vi "Page_Info_Initialize.vi"(8 "error in (no error)":errorcluster, 9 "ctlReferences":T1, 11 "AB_InteropAssembly in":refnum<class "AB_InteropAssembly.lvclass">) -> (0 "error out":errorcluster, 3 "AB_InteropAssembly out":refnum<class "AB_InteropAssembly.lvclass">)   [LabVIEW 2020, in "AB_InteropAssembly.lvclass"]
uses:
  <vilib>/AppBuilder/AB_Classes/InteropAssembly/AB_InteropAssembly.lvclass
  <resource>/Framework/Providers/Builds/AppBuilder/AB_UI_Page_Info_References.ctl
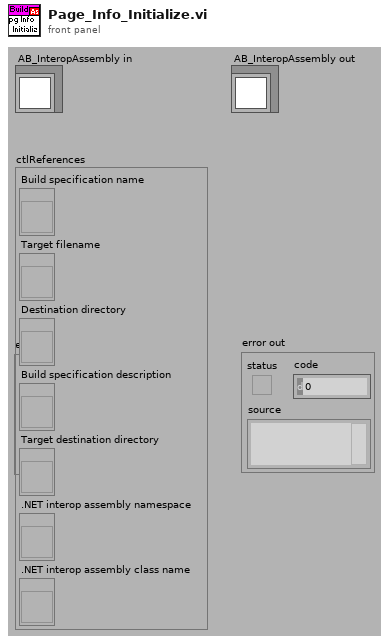
[diagram p1: front panel]
types:
  T1 = typedef "AB_UI_Page_Info_References.ctl" = cluster{"Build specification name":refnum<vi>, "Target filename":refnum<vi>, "Destination directory":refnum<vi>, "Build specification description":refnum<vi>, "Target destination directory":refnum<vi>, ".NET interop assembly namespace":refnum<vi>, ".NET interop assembly class name":refnum<vi>}
  T2 = typedef "LVRectTypeDef.ctl" = cluster{"Left":i16, "Top":i16, "Right":i16, "Bottom":i16}
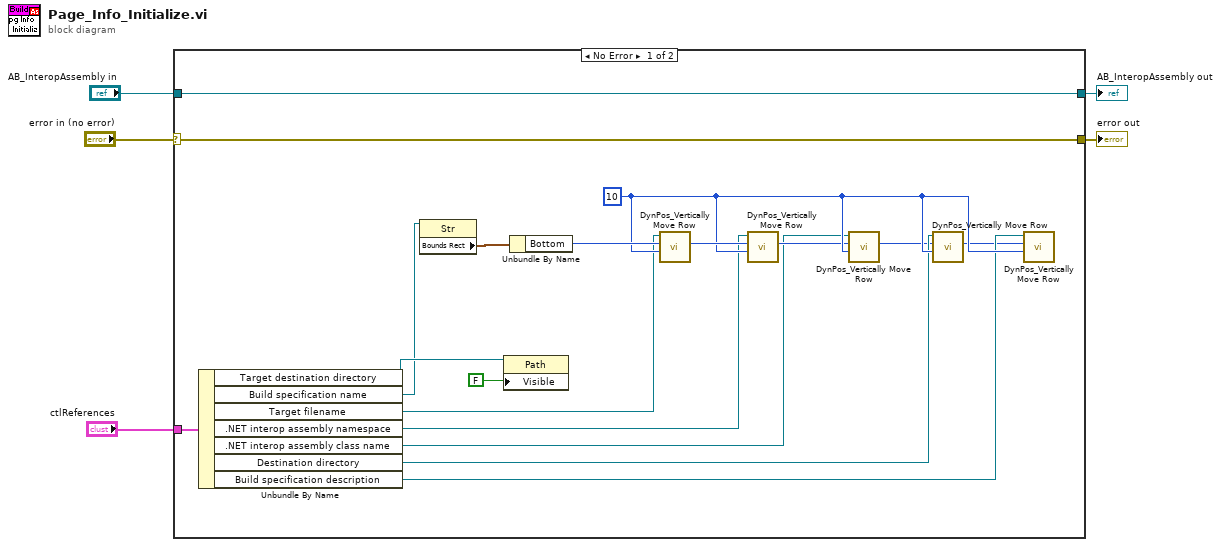
[diagram p0: block diagram]
diagram:
  n1 = case shown="No Error" "error in (no error)" {
    selector: "error in (no error)" -> [w6 w25]
    tunnel: [w6 w25] -> w1
    tunnel: [w7 w24] -> w4
    tunnel: "AB_InteropAssembly in" -> [w7 w24]
    tunnel: "ctlReferences" -> [w16 _]
    frame No Error {
      w17 = 10 ("Pixel separation (6)")
      n2 = Unbundle By Name(w16) -> ("Target destination directory"=w19:refnum<vi>, "Build specification name"=w18:refnum<vi>, "Target filename"=w13:refnum<vi>, ".NET interop assembly namespace"=w8:refnum<vi>, ".NET interop assembly class name"=w9:refnum<vi>, "Destination directory"=w14:refnum<vi>, "Build specification description"=w15:refnum<vi>)
      n3 = property class="Str"(reference=w18) -> ("Bounds Rect"=w23:T2)  [unwired: 1 in, 2 out]
      n4 = property class="Path"(reference=w19, "Visible"=FALSE) -> ()  [unwired: 1 in, 2 out]
      n5 = Unbundle By Name(w23) -> ("Bottom"=w22:i16)
      n6 = call <vilib>:"DynPos_Vertically Move Row.vi"("Pixel separation (6)"=w17, "Bottom of last control"=w22, "Control"=w13) -> ("Bottom pixel"=w21:i32)  [unwired: 1 in, 7 out]
      n7 = call <vilib>:"DynPos_Vertically Move Row.vi"("Pixel separation (6)"=w17, "Bottom of last control"=w21, "Control"=w8) -> ("Bottom pixel"=w12:i32)  [unwired: 1 in, 7 out]
      n8 = call <vilib>:"DynPos_Vertically Move Row.vi"("Pixel separation (6)"=w17, "Bottom of last control"=w12, "Control"=w9) -> ("Bottom pixel"=w11:i32)  [unwired: 1 in, 7 out]
      n9 = call <vilib>:"DynPos_Vertically Move Row.vi"("Pixel separation (6)"=w17, "Bottom of last control"=w11, "Control"=w14) -> ("Bottom pixel"=w10:i32)  [unwired: 1 in, 7 out]
      n10 = call <vilib>:"DynPos_Vertically Move Row.vi"("Pixel separation (6)"=w17, "Bottom of last control"=w10, "Control"=w15) -> ()  [unwired: 1 in, 8 out]
    }
    frame Error {
    }
  }
  "error out" <- w1
  "AB_InteropAssembly out" <- w4
